vi "ASYNC_Adam_client.vi"(2 "Values":dbl[](array[numeric]) format="%.2f", 3 "Check Value is in the scan table?":bool, 4 "Channel Names":string[](array[string])) -> (0 "Scan Comments":string[](array[string]), 1 "Calibrated Units":dbl[](array[numeric]) format="%.4f")   [LabVIEW 2021]
uses:
  Anemometry/Anemometry Sub Vis/Controls/Global_mode.ctl
  Sub VIs/ADAM Controls/Update_scan_value.ctl
  Anemometry/Anemometry Sub Vis/Globals/Preference_global.vi
panel:
  out "Iterations":i32
  in  "ASYNC Adam server":refnum<vi>
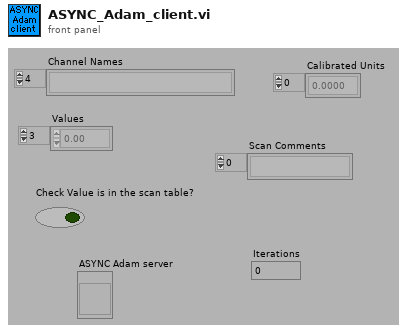
[diagram p1: front panel]
types:
  T1 = typedef "Server_Comms.ctl" = enum16{"Do Not Link To Server", "Server Link Healthy"}
  T2 = typedef "Update_scan_value.ctl" = cluster{"Channel Name":string, "New Value":dbl, "!Auto_Off":bool}
  T3 = typedef "Global_mode.ctl" = enum16{"Read Global", "Load Global From File", "Write Global to File"}
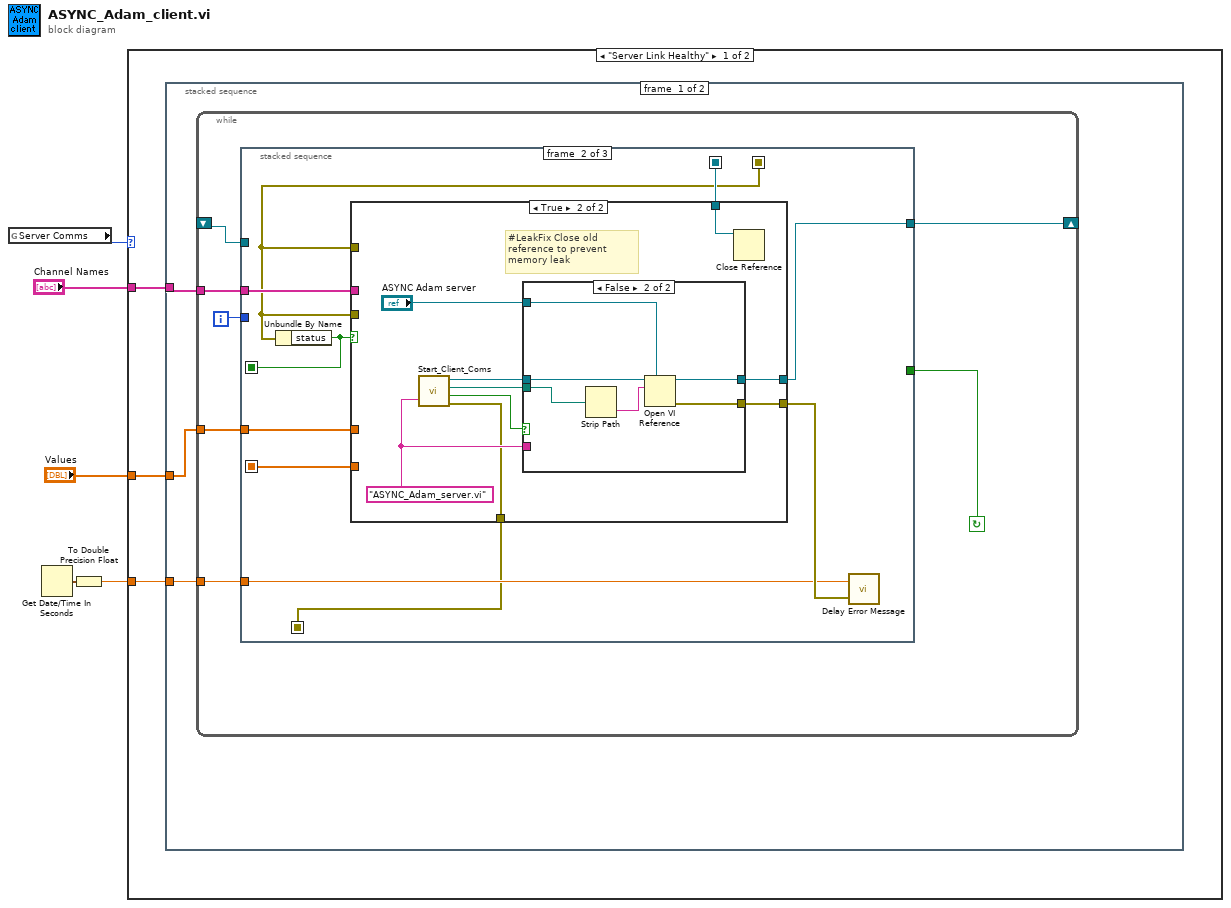
[diagram p0: block diagram]
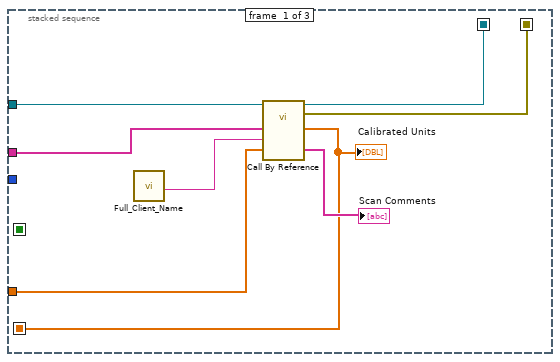
[diagram p2: hidden frame]
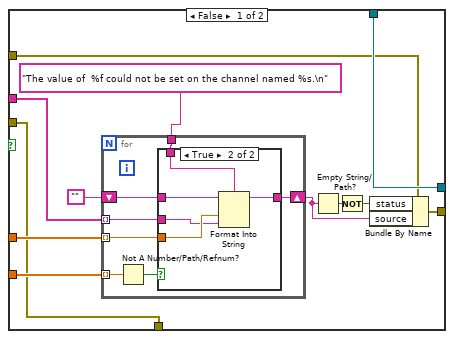
[diagram p3: hidden frame]
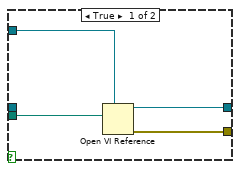
[diagram p5: hidden frame]
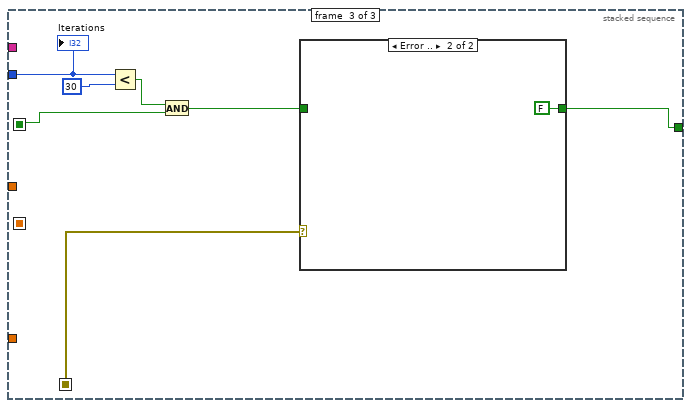
[diagram p6: hidden frame]
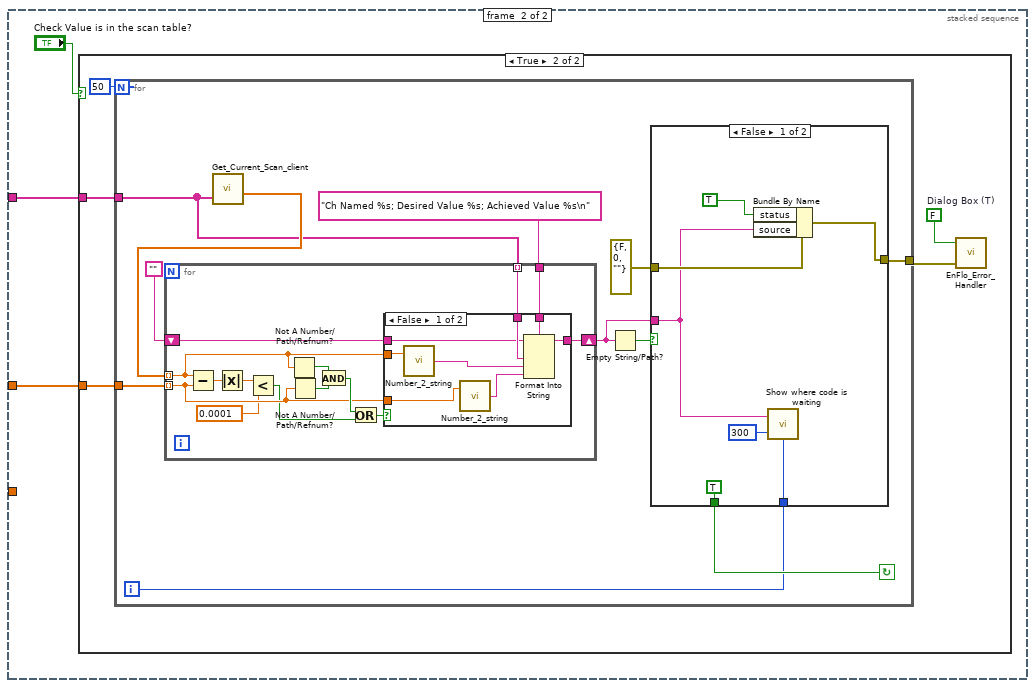
[diagram p8: hidden frame]
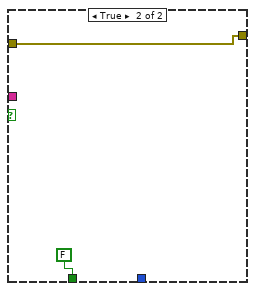
[diagram p11: hidden frame]
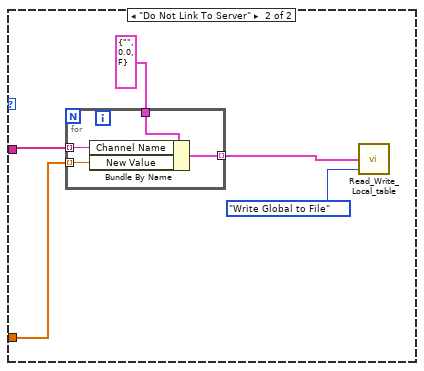
[diagram p12: hidden frame]
diagram:
  n1 = global read "Preference_global.vi" "Server Comms"() -> (w5:T1)
  n2 = Get Date/Time In Seconds() -> (seconds since 1Jan1904=w2:timestamp)
  n3 = To Double Precision Float(number=w2) -> (double precision float=w1:dbl)
  n4 = case shown="\"Server Link Healthy\"" w5 {
    tunnel: "Channel Names" -> [w8 w143]
    tunnel: "Values" -> [w7 w142]
    tunnel: w1 -> [w6 _]
    frame "Server Link Healthy" {
      n5 = stacked-sequence {
        tunnel: w8 -> [w11 w91]
        tunnel: w7 -> [w10 w90]
        tunnel: w6 -> [w9 _]
        frame #0 {
          n6 = while {
            tunnel: w10 -> [w13]
            tunnel: w11 -> [w14]
            shift-left: _ -> [w18]
            shift-right: [w17] -> _
            tunnel: w9 -> [w12]
            i -> [w16]
            stop <- w15 continue-if-true
            n7 = stacked-sequence {
              seq-local: [w24 _ _] -> [_ w36 _]
              seq-local: [w26 _ _] -> [_ w27 _]
              seq-local: [_ w35 _] -> [_ _ w84]
              seq-local: [w19 _ _] -> [_ w33 _]
              seq-local: [_ w28 _] -> [_ _ w83]
              tunnel: w18 -> [w25 _ _]
              tunnel: [_ w34 _] -> w17
              tunnel: w16 -> [_ _ w85]
              tunnel: [_ _ w82] -> w15
              tunnel: w14 -> [w22 w31 _]
              tunnel: w13 -> [w21 w32 _]
              tunnel: w12 -> [_ w29 _]
              frame #0 {
                n8 = call "Full_Client_Name.vi"() -> ("Client Name"=w20:string)
                n9 = call-by-ref "?"(reference=w25, "Values"=w21, "Client Name"=w20, "Channel Names"=w22) -> (reference out=w24:refnum<vi>, error out=w26:errorcluster, "Scan Comments"=→"Scan Comments":string[], "Calibrated Units"=w19:dbl[])  [unwired: 2 in]
                "Calibrated Units" <- w19
              }
              frame #1 {
                n10 = Unbundle By Name(w27) -> ("status"=w35:bool)
                n11 = case shown="True" w35 {
                  tunnel: w36 -> [w48 w63]
                  tunnel: [w41 w67] -> w30
                  tunnel: w27 -> [w42 _]
                  tunnel: [w48 w66] -> w34
                  tunnel: w33 -> [w47 _]
                  tunnel: w32 -> [w46 _]
                  tunnel: w31 -> [w45 _]
                  tunnel: [w37 w62] -> w28
                  tunnel: w27 -> [w37 _]
                  frame False {
                    n12 = for {
                      shift-right: [w50] -> w38
                      shift-left: "" -> [w51]
                      tunnel: w47 -> [w55] mode=indexing
                      tunnel: w46 -> [w53] mode=indexing
                      tunnel: w45 -> [w52] mode=indexing
                      tunnel: "The value of  %f could not be set on the channel named %s.\n" ("format string") -> [w49]
                      n13 = Not A Number/Path/Refnum?(number/path/refnum=w55) -> (NaN/Path/Refnum?=w54:bool)
                      n14 = case shown="True" w54 {
                        tunnel: w53 -> [_ w61]
                        tunnel: w52 -> [_ w60]
                        tunnel: w51 -> [w56 w59]
                        tunnel: [w56 w58] -> w50
                        tunnel: w49 -> [_ w57]
                        frame False {
                        }
                        frame True {
                          n15 = Format Into String(format string=w57, initial string=w59, w61, w60) -> (resulting string=w58:string)  [unwired: 1 in, 1 out]
                        }
                      }
                    }
                    n16 = Empty String/Path?(string/path=w38) -> (empty?=w40:bool)
                    n17 = Not(x=w40) -> (.not. x?=w39:bool)
                    n18 = Bundle By Name(cluster=w42, "status"=w39, "source"=w38) -> (w41:errorcluster)
                  }
                  frame True {
                    w65 = "ASYNC_Adam_server.vi"
                    # "#LeakFix Close old reference to prevent memory leak"
                    n19 = call "Start_Client_Coms.vi"("VI name to run on server"=w65) -> ("LabVIEW application reference"=w70:refnum<vi>, "Checked VI name"=w68:path, "Local Call"=w69:bool, "Error cluster"=w62:errorcluster)  [unwired: 1 in]
                    n20 = case shown="False" w69 {
                      tunnel: w68 -> [w74 w77]
                      tunnel: w70 -> [_ w75]
                      tunnel: [w73 w78] -> w67
                      tunnel: [w72 w79] -> w66
                      tunnel: w65 -> [_ _]
                      tunnel: "ASYNC Adam server" -> [w71 w76]
                      frame True {
                        n21 = Open VI Reference(type specifier VI Refnum (for type only)=w71, vi path=w74) -> (vi reference=w72:refnum<vi>, error out=w73:errorcluster)  [unwired: 1 in, 3 out]
                      }
                      frame False {
                        n22 = Strip Path(path=w77) -> (name=w80:string)  [unwired: 1 out]
                        n23 = Open VI Reference(type specifier VI Refnum (for type only)=w76, application reference (local)=w75, vi path=w80) -> (vi reference=w79:refnum<vi>, error out=w78:errorcluster)  [unwired: 1 in, 2 out]
                      }
                    }
                    n24 = Close Reference(reference=w63) -> ()  [unwired: 1 in, 1 out]
                  }
                }
                n25 = call "Delay Error Message.vi"("error in (no error)"=w30, "Seconds since 1904"=w29) -> ()  [unwired: 2 in]
              }
              frame #2 {
                n26 = Less?(x=w85, y=30) -> (x < y?=w87:bool)
                n27 = And(x=w87, y=w84) -> (x .and. y?=w81:bool)
                n28 = case shown="Error .." w83 {
                  tunnel: [w88 FALSE] -> w82
                  tunnel: w81 -> [w88 _]
                  frame No Error {
                  }
                  frame Error {
                  }
                }
                "Iterations" <- w85
              }
            }
          }
        }
        frame #1 {
          n29 = case shown="True" "Check Value is in the scan table?" {
            tunnel: w91 -> [_ w96]
            tunnel: w90 -> [_ w95]
            frame False {
            }
            frame True {
              w94 = FALSE  # Dialog Box (T)
              n30 = for {
                N: 50 -> [_]
                tunnel: w96 -> [w104]
                tunnel: w95 -> [w105]
                tunnel: [w100] -> w93
                i -> [w98]
                stop <- w101 continue-if-true
                n31 = call "Get_Current_Scan_client.vi"("multipleChannels"=w104) -> ("Numerical Values"=w106:dbl[])  [unwired: 1 in, 3 out]
                n32 = for {
                  shift-right: [w121] -> w102
                  shift-left: "" -> [w120]
                  tunnel: w105 -> [w113] mode=indexing
                  tunnel: w106 -> [w114] mode=indexing
                  tunnel: "Ch Named %s; Desired Value %s; Achieved Value %s\n" ("format string") -> [w122]
                  tunnel: w104 -> [w115] mode=indexing
                  n33 = Subtract(x=w114, y=w113) -> (x-y=w112:dbl)
                  n34 = Absolute Value(x=w112) -> (abs(x)=w111:dbl)
                  n35 = Less?(x=w111, y=0.0001) -> (x < y?=w109:bool)
                  n36 = Not A Number/Path/Refnum?(number/path/refnum=w114) -> (NaN/Path/Refnum?=w117:bool)
                  n37 = Not A Number/Path/Refnum?(number/path/refnum=w113) -> (NaN/Path/Refnum?=w118:bool)
                  n38 = And(x=w117, y=w118) -> (x .and. y?=w116:bool)
                  n39 = Or(x=w116, y=w109) -> (x .or. y?=w119:bool)
                  n40 = case shown="False" w119 {
                    tunnel: w115 -> [w130 _]
                    tunnel: w114 -> [w124 _]
                    tunnel: w113 -> [w125 _]
                    tunnel: w122 -> [w123 _]
                    tunnel: [w129 w131] -> w121
                    tunnel: w120 -> [w128 w131]
                    frame False {
                      n41 = call "Number_2_string.vi"("number"=w124) -> ("String"=w126:string)  [unwired: 1 in]
                      n42 = call "Number_2_string.vi"("number"=w125) -> ("String"=w127:string)  [unwired: 1 in]
                      n43 = Format Into String(format string=w123, initial string=w128, w130, w126, w127) -> (resulting string=w129:string)  [unwired: 1 in, 1 out]
                    }
                    frame True {
                    }
                  }
                }
                n44 = Empty String/Path?(string/path=w102) -> (empty?=w103:bool)
                n45 = case shown="False" w103 {
                  tunnel: [TRUE FALSE] -> w101
                  tunnel: w102 -> [w132 _]
                  tunnel: [w138 w139] -> w100
                  tunnel: errorcluster {"status"=FALSE, "code"=0, "source"=""} ("error in (no error)") -> [w135 w139]
                  tunnel: w98 -> [w133 _]
                  frame False {
                    n46 = Bundle By Name(cluster=w135, "status"=TRUE, "source"=w132) -> (w138:errorcluster)
                    n47 = call "Show where code is waiting.vi"("Loop index"=w133, "Wait (ms)"=u32 300 ("milliseconds to wait"), "Message"=w132) -> ()  [unwired: 1 in]
                  }
                  frame True {
                  }
                }
              }
              n48 = call "EnFlo_Error_Handler.vi"("error in (no error)"=w93, "Dialog Box (F)"=w94) -> ()  [unwired: 1 in, 3 out]
            }
          }
        }
      }
    }
    frame "Do Not Link To Server" {
      n49 = for {
        tunnel: T2 {"Channel Name"="", "New Value"=0.0, "!Auto_Off"=FALSE} ("Update Scan Value Cluster") -> [w149]
        tunnel: w143 -> [w148] mode=indexing
        tunnel: w142 -> [w147] mode=indexing
        tunnel: [w146] -> w141 mode=indexing
        n50 = Bundle By Name(cluster=w149, "Channel Name"=w148, "New Value"=w147) -> (w146:T2)
      }
      n51 = call "Read_Write_Local_table.vi"("Mode"=Global_mode."Write Global to File", "Ch Values in"=w141) -> ()  [unwired: 1 in, 3 out]
    }
  }
